vi "VisaReadforPumps.vi"(8 "error in (no error)":errorcluster, 10 "Byte Count":i32, 11 "VISA Refnum in":refnum<visa-resource-name>) -> (0 "error out":errorcluster, 1 "Read (Response)":string, 2 "Read (BLANK)":string, 3 "VISA Refnum out":refnum<visa-resource-name>)   [LabVIEW 2014]
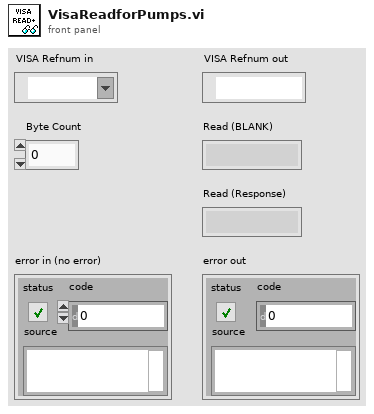
[diagram p1: front panel]
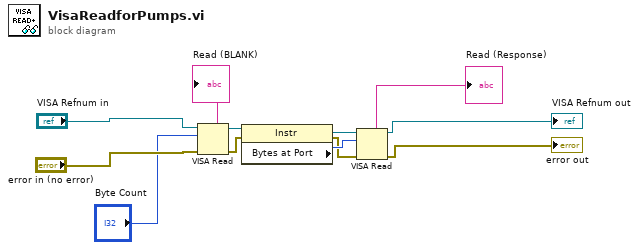
[diagram p0: block diagram]
diagram:
  n1 = VISA Read(VISA resource name="VISA Refnum in", byte count="Byte Count", error in (no error)="error in (no error)") -> (VISA resource name out=w5:refnum<visa-resource-name>, read buffer=→"Read (BLANK)":string, error out=w6:errorcluster)  [unwired: 1 out]
  n2 = property class="Instr"(reference=w5, error in=w6) -> (reference out=w7:refnum<visa-resource-name>, error out=w8:errorcluster, "Bytes at Port"=w9:u32)
  n3 = VISA Read(VISA resource name=w7, byte count=w9, error in (no error)=w8) -> (VISA resource name out=→"VISA Refnum out":refnum<visa-resource-name>, read buffer=→"Read (Response)":string, error out=→"error out":errorcluster)  [unwired: 1 out]
